vi "Handle setConfiguration.vi"(8 "error in (no error)":errorcluster, 10 "setConfiguration":variant, 11 "Instrument.FrameworkTemplate":refnum<class "Instrument.FrameworkTemplate.lvclass">) -> (0 "error out":errorcluster, 3 "Instrument.FrameworkTemplate out":refnum<class "Instrument.FrameworkTemplate.lvclass">)   [LabVIEW 2019, in "Instrument.FrameworkTemplate.lvclass"]
uses:
  Instrument.FrameworkTemplate.lvclass
  Instrument.FrameworkTemplate.lvclass/Instrument.FrameworkTemplate.ctl
  7fd627c4-46b3-46d4-9a3c-07d9147c5e06.vi
  7fd627c4-46b3-46d4-9a3c-07d9147c5e06.vi/d3f07ac4-ac26-448c-b218-0b28afc030e1.vi
  7fd627c4-46b3-46d4-9a3c-07d9147c5e06.vi/ecb76ffe-1ebe-4b28-8dfb-e8527a989120.vi
  <vilib>/JDP Science/JSONtext/JSON text to Variant.vi
  <vilib>/JDP Science/JSONtext/LVClass Serializer/JSONtext LVClass Serializer.lvclass
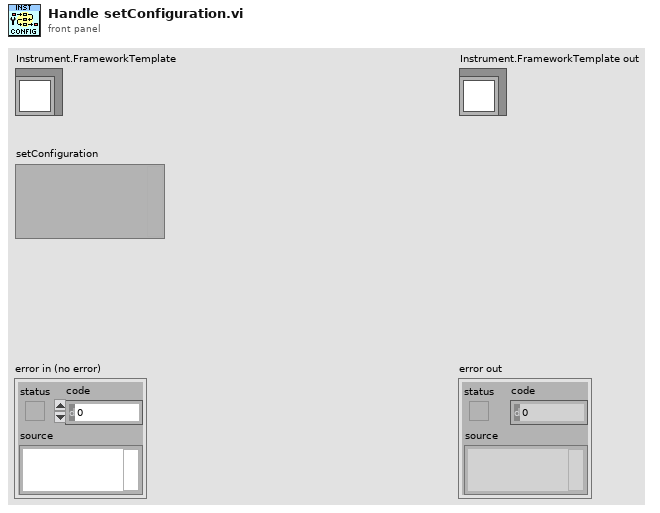
[diagram p1: front panel]
types:
  T1 = typedef "Instrument.FrameworkTemplate.lvclass/Instrument.FrameworkTemplate.Configuration--Cluster.ctl" = cluster{"Example Setting 1":dbl, "Example Setting 2":dbl, "Example Setting 3":string}
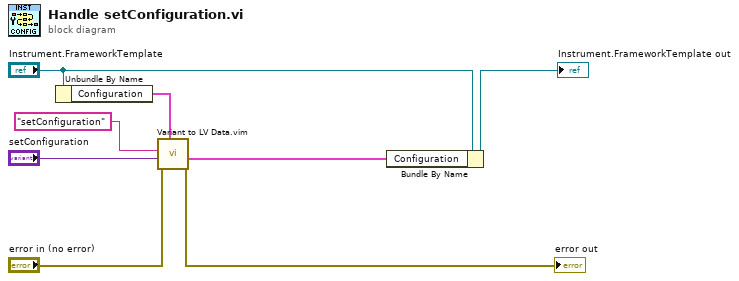
[diagram p0: block diagram]
diagram:
  n1 = Unbundle By Name("Instrument.FrameworkTemplate") -> ("Configuration"=w7:T1)
  n2 = call "Variant to LV Data.vim"("type"=w7, "error in (no error)"="error in (no error)", "Data in"="setConfiguration", "Command"="setConfiguration") -> ("error out"=→"error out":errorcluster, "Data out"=w1:T1)  [unwired: 4 in, 2 out]
  n3 = Bundle By Name(cluster="Instrument.FrameworkTemplate", "Configuration"=w1) -> (→"Instrument.FrameworkTemplate out":refnum<class "Instrument.FrameworkTemplate.lvclass">)
